vi "LeftLeft.vi"   [LabVIEW 2017]
types:
  T1 = typedef "Command Status Info.ctl" = cluster{"Name":string, "Status":T2, "notifier out":T3}
  T2 = typedef "Completion Status.ctl" = enum16{"Successful", "Aborted", "Incomplete"}
  T3 = typedef "Completion Notifier.ctl" = refnum<notifier>
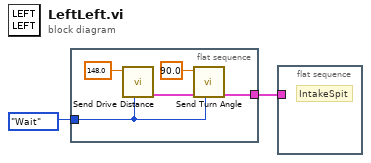
[diagram p0: block diagram]
diagram:
  n1 = flat-sequence {
    tunnel: [w5] -> w1
    tunnel: enum16{"Start", "Wait"}."Wait" ("Synchronization") -> [w3]
    frame #0 {
      n2 = call "Send Drive Distance.vi"("Synchronization"=w3, "Target Distance"=148.0) -> ("Command Info Out"=w4:T1)  [unwired: 8 in, 1 out]
      n3 = call "Send Turn Angle.vi"("Synchronization"=w3, "Command Info In"=w4, "Target Angle"=90.0) -> ("Command Info Out"=w5:T1)  [unwired: 7 in, 1 out]
    }
  }
  n4 = flat-sequence {
    tunnel: w1 -> [_]
    frame #0 {
      # "IntakeSpit"
    }
  }
